vi "caseChoicePassTest.vi"(8 "Out of the field":T1, 9 "Ball stops":T1, 10 "Pass intercepted":T1, 11 "Too much force\nCorrect pass\nKeep ball possesion\nInvalid Situation\nPass on the way":T1) -> (3 "Result":T1)   [LabVIEW 2018]
uses:
  passTestStates.ctl
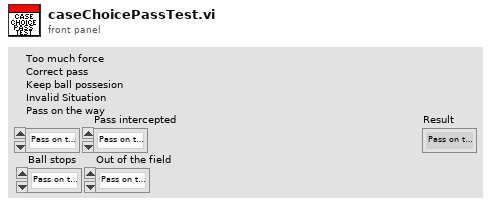
[diagram p1: front panel]
types:
  T1 = typedef "passTestStates.ctl" = enum16{"Pass on the way", "Ball stops", "Pass intercepted", "Ball out of the field", "Ball missed robot", "Need more force to pass", "Too much force", "Correct pass", "Keep ball possesion", "Robot kicked the ball", "Waiting Kick", "Invalid: same robot", "Invalid: kicker ID 999", "Invalid: Receiver ID 999", "Invalid"}
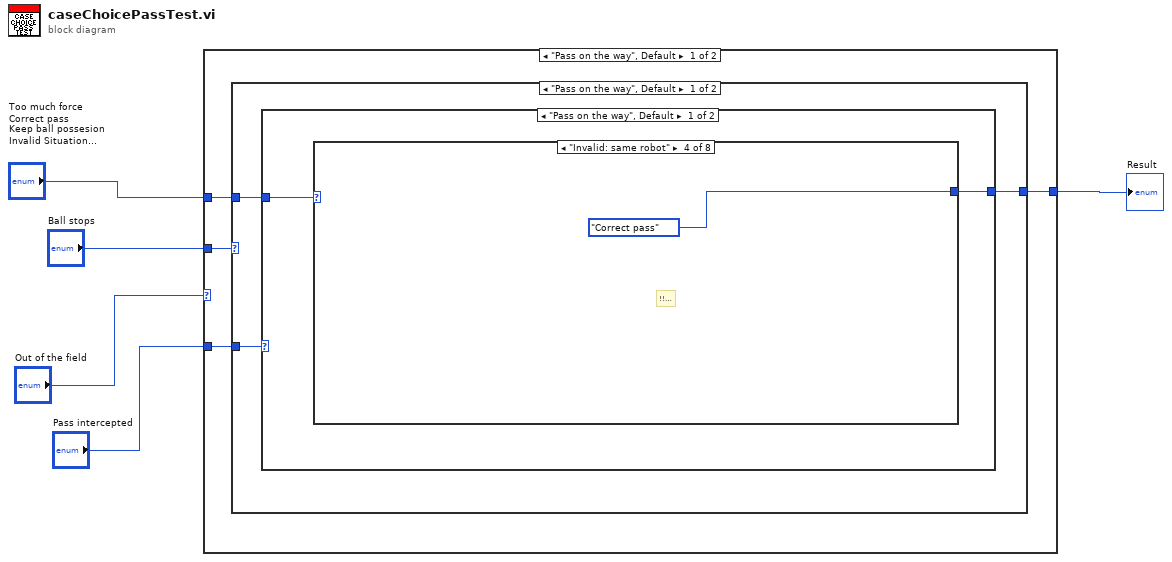
[diagram p0: block diagram]
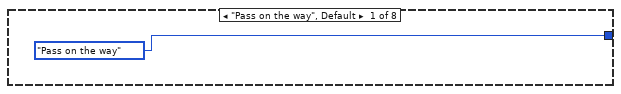
[diagram p2: hidden frame]
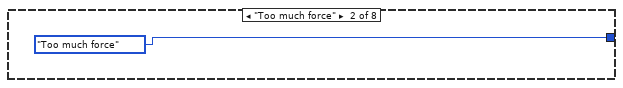
[diagram p3: hidden frame]
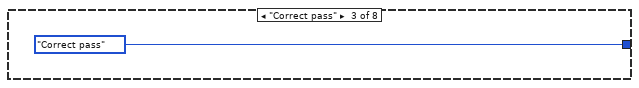
[diagram p4: hidden frame]
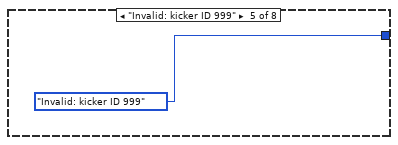
[diagram p5: hidden frame]
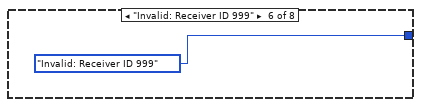
[diagram p6: hidden frame]
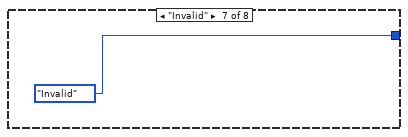
[diagram p7: hidden frame]
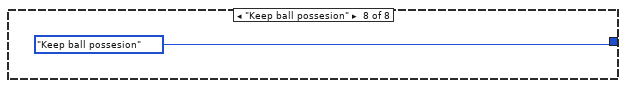
[diagram p8: hidden frame]
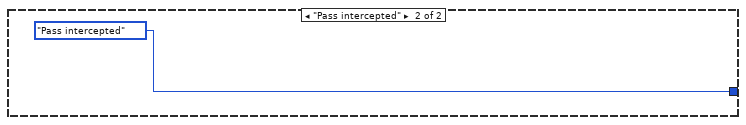
[diagram p9: hidden frame]
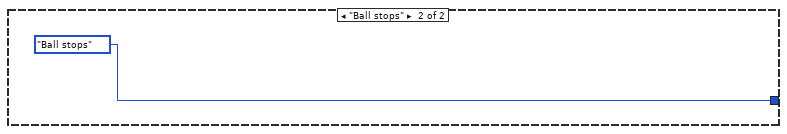
[diagram p10: hidden frame]
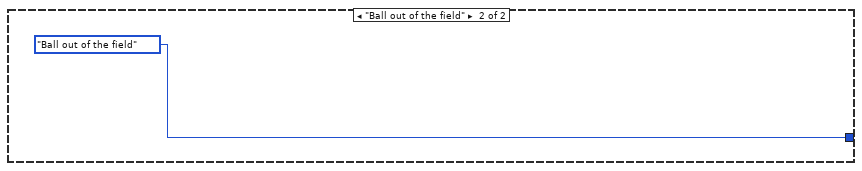
[diagram p11: hidden frame]
diagram:
  n1 = case shown="\"Pass on the way\", Default" "Out of the field" {
    tunnel: "Ball stops" -> [w9 _]
    tunnel: "Pass intercepted" -> [w8 _]
    tunnel: "Too much force\nCorrect pass\nKeep ball possesion\nInvalid Situation\nPass on the way" -> [w7 _]
    tunnel: [w6 passTestStates."Ball out of the field"] -> w1
    frame "Pass on the way", Default {
      n2 = case shown="\"Pass on the way\", Default" w9 {
        tunnel: w8 -> [w12 _]
        tunnel: w7 -> [w11 _]
        tunnel: [w10 passTestStates."Ball stops"] -> w6
        frame "Pass on the way", Default {
          n3 = case shown="\"Pass on the way\", Default" w12 {
            tunnel: w11 -> [w14 _]
            tunnel: [w13 passTestStates."Pass intercepted"] -> w10
            frame "Pass on the way", Default {
              n4 = case shown="\"Invalid: same robot\"" w14 {
                tunnel: [passTestStates."Pass on the way" passTestStates."Too much force" passTestStates."Correct pass" passTestStates."Correct pass" passTestStates."Invalid: kicker ID 999" passTestStates."Invalid: Receiver ID 999" passTestStates."Invalid" passTestStates."Keep ball possesion"] -> w13
                frame "Pass on the way", Default {
                }
                frame "Too much force" {
                }
                frame "Correct pass" {
                }
                frame "Invalid: same robot" {
                  # "!!!!!"
                }
                frame "Invalid: kicker ID 999" {
                }
                frame "Invalid: Receiver ID 999" {
                }
                frame "Invalid" {
                }
                frame "Keep ball possesion" {
                }
              }
            }
            frame "Pass intercepted" {
            }
          }
        }
        frame "Ball stops" {
        }
      }
    }
    frame "Ball out of the field" {
    }
  }
  "Result" <- w1
